vi "bool-test.vi"(11 "布尔":bool) -> (3 "布尔 2":bool)   [LabVIEW 2020]
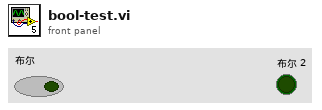
[diagram p1: front panel]
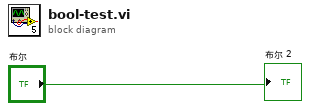
[diagram p0: block diagram]
diagram:
  "布尔 2" <- "布尔"
